vi "AUTON_Unpack.vi"(0 "all rows":dbl[][](array[numeric]), 5 "Index":i32) -> (4 "Primitive ID":i16, 6 "Desired Heading":dbl, 8 "Time/Distance":dbl, 10 "Power":dbl, 13 "Moved":dbl, 14 "Shoot":dbl, 15 "Harvest":dbl)   [LabVIEW 2013]
doc: "Use this VI to separate the autonomous array data into individual arrays. First array is Primitive ID, second is heading, etc."
panel:
  out "Misc 4":dbl
  out "Misc 3":dbl
  out "Misc 2":dbl
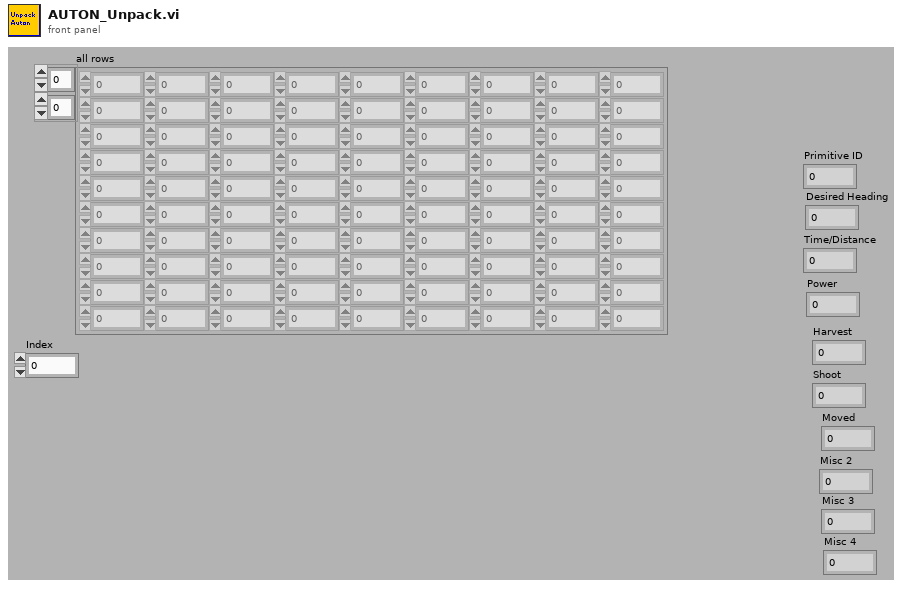
[diagram p1: front panel]
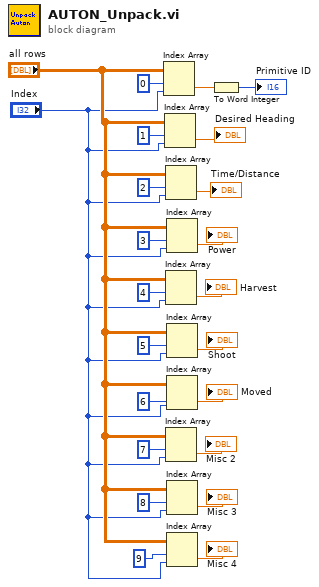
[diagram p0: block diagram]
diagram:
  n1 = Index Array(array="all rows", index (row)=0, index (col)="Index") -> (element=w20:dbl)
  n2 = Index Array(array="all rows", index (row)=1, index (col)="Index") -> (element=→"Desired Heading":dbl)
  n3 = Index Array(array="all rows", index (row)=2, index (col)="Index") -> (element=→"Time/Distance":dbl)
  n4 = Index Array(array="all rows", index (row)=4, index (col)="Index") -> (element=→"Harvest":dbl)
  n5 = Index Array(array="all rows", index (row)=7, index (col)="Index") -> (element=→"Misc 2":dbl)
  n6 = Index Array(array="all rows", index (row)=3, index (col)="Index") -> (element=→"Power":dbl)
  n7 = Index Array(array="all rows", index (row)=5, index (col)="Index") -> (element=→"Shoot":dbl)
  n8 = Index Array(array="all rows", index (row)=6, index (col)="Index") -> (element=→"Moved":dbl)
  n9 = Index Array(array="all rows", index (row)=8, index (col)="Index") -> (element=→"Misc 3":dbl)
  n10 = Index Array(array="all rows", index (row)=9, index (col)="Index") -> (element=→"Misc 4":dbl)
  n11 = To Word Integer(number=w20) -> (16bit integer=→"Primitive ID":i16)
